vi "Edit Configuration.vi"(8 "error in (no error)":errorcluster, 11 "Ports to Check":T1) -> (0 "error out":errorcluster, 3 "Ports to Check":T1)   [LabVIEW 2019]
doc: "This VI edits the configuration file local to this instance of the application. The ports to check are specified here."
uses:
  controls/Ports to Check.ctl
  <vilib>/Utility/config.llb/Write Key (U32).vi
  <vilib>/Utility/config.llb/NI_LVConfig.lvlib
panel:
  in  "InsightCM Defaults":bool
  in  "OK Button":bool
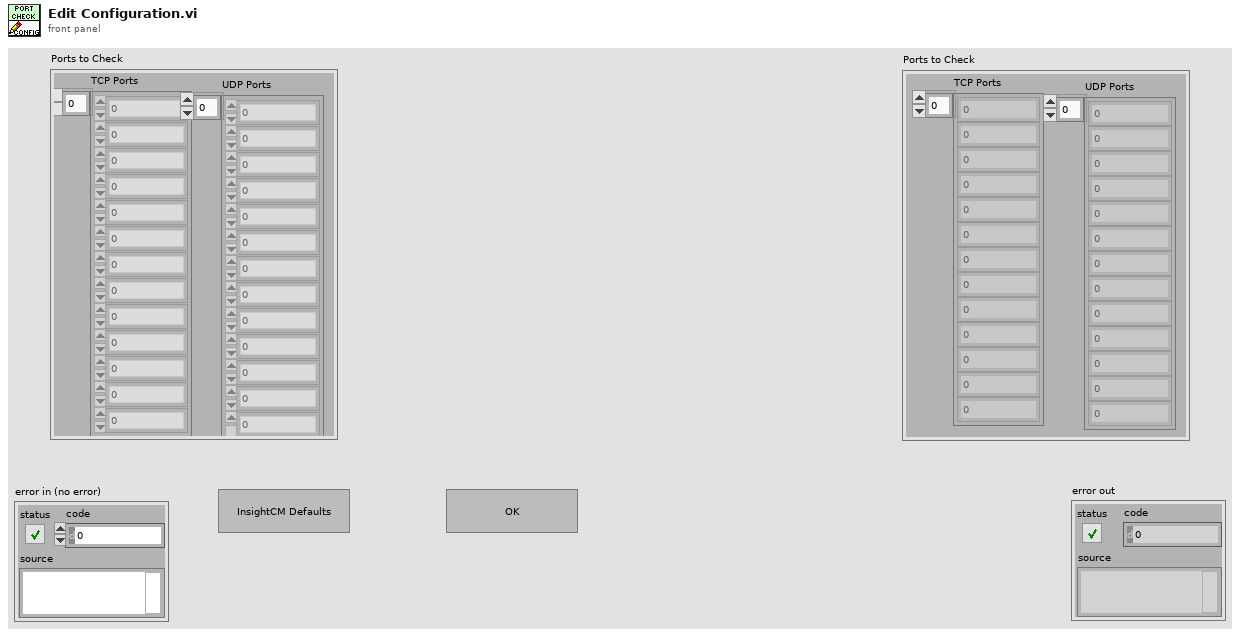
[diagram p1: front panel]
types:
  T1 = typedef "Ports to Check.ctl" = cluster{"TCP Ports":u32[], "UDP Ports":u32[]}
  T2 = typedef "NI_LVConfig.lvlib/Config Data RefNum.ctl" = refnum<k1>
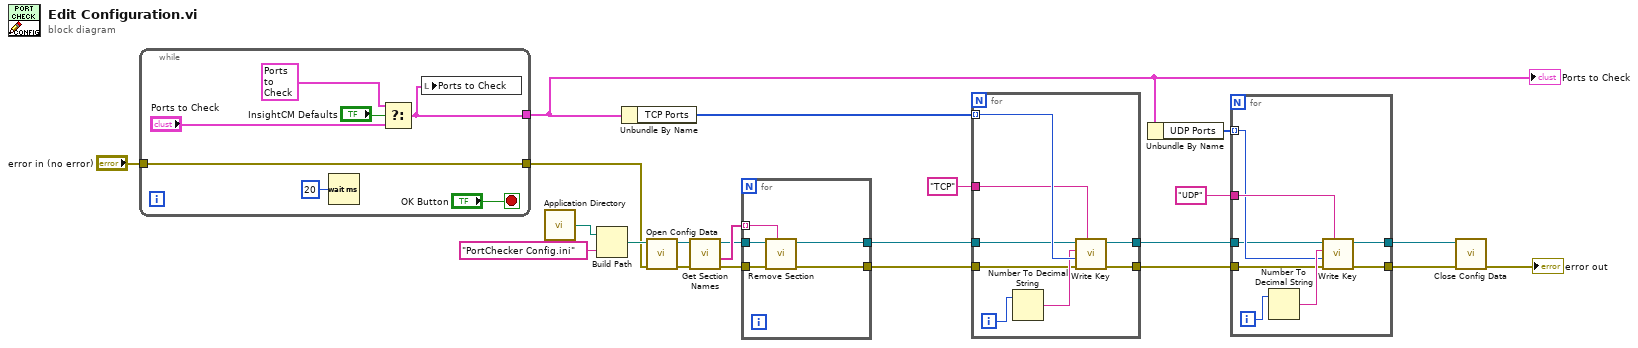
[diagram p0: block diagram]
diagram:
  n1 = while {
    tunnel: "error in (no error)" -> [w28]
    tunnel: [w28] -> w15
    tunnel: [w23] -> w1
    stop <- "OK Button" stop-if-true
    n2 = Wait (ms)(milliseconds to wait=u32 20) -> ()  [unwired: 1 out]
    n3 = Select(t=T1 {"TCP Ports"=[82, 482, 5672, 6343, 8002, 49580, 3580, 80, 22, 44516, 52725, 8080], "UDP Ports"=[5353, 44515, 44525]} ("Ports to Check"), s="InsightCM Defaults", f="Ports to Check") -> (s? t:f=w23:T1)
    n4 = local write "Ports to Check"(w23) -> ()
  }
  "Ports to Check" <- w1
  n5 = call <vilib>:"Application Directory.vi"() -> ("Application Directory"=w21:path)
  n6 = Build Path(base path=w21, name or relative path="PortChecker Config.ini") -> (appended path=w19:path)
  n7 = Unbundle By Name(w1) -> ("TCP Ports"=w18:u32[])
  n8 = call <vilib>:"Open Config Data.vi"("error in (no error)"=w15, "configuration file path"=w19) -> ("error out"=w8:errorcluster, "refnum"=w7:T2)  [unwired: 7 in, 1 out]
  n9 = call <vilib>:"Get Section Names.vi"("error in (no error)"=w8, "refnum"=w7) -> ("error out"=w4:errorcluster, "section names"=w6:string[], "refnum out"=w5:T2)  [unwired: 7 in]
  n10 = for {
    tunnel: w6 -> [w34] mode=indexing
    tunnel: w5 -> [w33]
    tunnel: w4 -> [w32]
    tunnel: [w31] -> w3
    tunnel: [w30] -> w2
    n11 = call <vilib>:"Remove Section.vi"("section"=w34, "error in (no error)"=w32, "refnum"=w33) -> ("error out"=w30:errorcluster, "refnum out"=w31:T2)  [unwired: 6 in, 1 out]
  }
  n12 = for {
    tunnel: w3 -> [w41]
    tunnel: w18 -> [w42] mode=indexing
    tunnel: "TCP" ("key") -> [w40]
    tunnel: [w37] -> w12
    tunnel: [w36] -> w11
    tunnel: w2 -> [w35]
    i -> [w39]
    n13 = Number To Decimal String(number=w39) -> (decimal integer string=w38:string)  [unwired: 1 in]
    n14 = call-poly <vilib>:"Write Key.vi"("section"=w40, "error in (no error)"=w35, "value"=w42, "key"=w38, "refnum"=w41) -> ("error out"=w36:errorcluster, "refnum out"=w37:T2)  [unwired: 4 in, 1 out]
  }
  n15 = Unbundle By Name(w1) -> ("UDP Ports"=w13:u32[])
  n16 = for {
    tunnel: "UDP" ("key") -> [w50]
    tunnel: w13 -> [w47] mode=indexing
    tunnel: w12 -> [w46]
    tunnel: w11 -> [w45]
    tunnel: [w44] -> w10
    tunnel: [w43] -> w9
    i -> [w49]
    n17 = Number To Decimal String(number=w49) -> (decimal integer string=w48:string)  [unwired: 1 in]
    n18 = call-poly <vilib>:"Write Key.vi"("section"=w50, "error in (no error)"=w45, "value"=w47, "key"=w48, "refnum"=w46) -> ("error out"=w44:errorcluster, "refnum out"=w43:T2)  [unwired: 4 in, 1 out]
  }
  n19 = call <vilib>:"Close Config Data.vi"("error in (no error)"=w10, "refnum"=w9) -> ("error out"=→"error out":errorcluster)  [unwired: 8 in, 1 out]
